vi "H5Pget_fclose_degree.vi"(6 "error in (no error)":errorcluster, 9 "HDF5 Property List Ref":T2) -> (0 "error out":errorcluster, 2 "Close degree":T1 items=["H5F_CLOSE_DEFAULT", "H5F_CLOSE_WEAK", "H5F_CLOSE_SEMI", "H5F_CLOSE_STRONG"], 3 "HDF5 Property List Ref out":T2)   [LabVIEW 2017]
doc: "Returns the file close degree."
uses:
  <vilib>/UPVI/lvhdf5/library.llb/HDF5 Ref.ctl
  <vilib>/UPVI/lvhdf5/property.llb/H5F_close_degree_t.ctl
  <vilib>/UPVI/lvhdf5/hdf5.dll
panel:
  # "LVHDF5 Toolkit\nCopyright (c) 2005-2013 by Jason D. Sommerville\nCopyright (c) 2014 by UPVI, LLC.\n\nThis use and distribution of this file is governed by the terms found in \nLICENSE.txt distributed with this toolkit and installed at\n <user.lib>\\_lvhdf5\\LICENSE.txt"
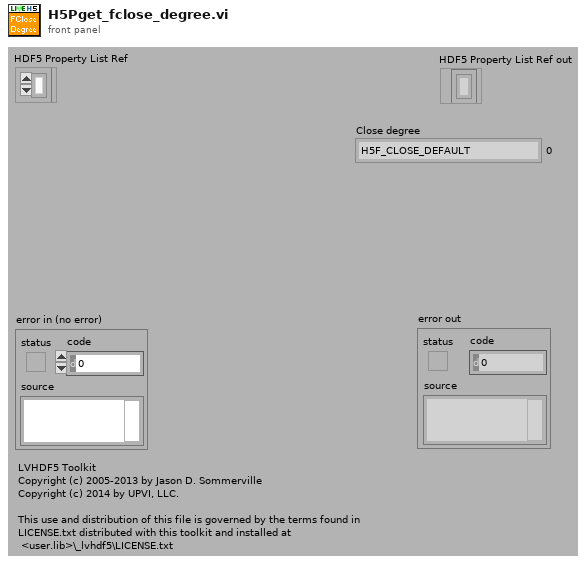
[diagram p1: front panel]
types:
  T1 = typedef "H5F_close_degree_t.ctl" = i32
  T2 = typedef "HDF5 Ref.ctl" = refnum<k1>
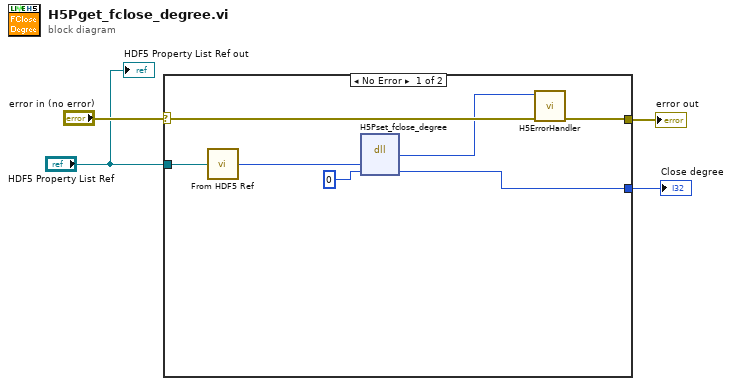
[diagram p0: block diagram]
diagram:
  n1 = case shown="No Error" "error in (no error)" {
    selector: "error in (no error)" -> [w11 w12]
    tunnel: [w10 w12] -> w3
    tunnel: "HDF5 Property List Ref" -> [w9 _]
    tunnel: [w5 _] -> w1
    frame No Error {
      n2 = call <vilib>:"From HDF5 Ref.vi"("HDF5 Ref"=w9) -> ("I32"=w8:i32)
      n3 = dll-call lib="C:/Program Files/National Instruments/LabVIEW 2017/vi.lib/UPVI/lvhdf5/hdf5.dll" fn="H5Pset_fclose_degree"("plist_id"=w8, "fc_degree"=0) -> (w7:i32, "fc_degree"=w5:i32)  [unwired: 4 in, 2 out]
      n4 = call <vilib>:"H5ErrorHandler.vi"("error in (no error)"=w11, "herr_t"=w7) -> ("error out"=w10:errorcluster)  [unwired: 3 in, 4 out]
    }
    frame Error {
    }
  }
  "error out" <- w3
  "Close degree" <- w1
  "HDF5 Property List Ref out" <- "HDF5 Property List Ref"
